vi "ex_BackUpExistFile.vi"(8 "error in":errorcluster, 11 "file path":path) -> (0 "error out":errorcluster, 3 "dup file path":path)   [LabVIEW 2017]
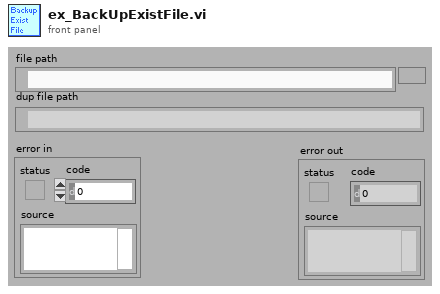
[diagram p1: front panel]
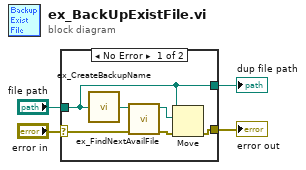
[diagram p0: block diagram]
diagram:
  n1 = case shown="No Error" "error in" {
    selector: "error in" -> [w10 w12]
    tunnel: [w6 w12] -> w3
    tunnel: "file path" -> [w5 w11]
    tunnel: [w5 w11] -> w1
    frame No Error {
      n2 = call <vilib>:"ex_CreateBackupName.vi"("original name"=w5) -> ("backup name"=w9:path)  [unwired: 4 out]
      n3 = call <vilib>:"ex_FindNextAvailFile.vi"("error in"=w10, "desired file path"=w9) -> ("error out"=w8:errorcluster, "next avail file path"=w7:path)  [unwired: 8 out]
      n4 = Move(source path=w5, error in=w8, 10:w7) -> (error out=w6:errorcluster)  [unwired: 4 out]
    }
    frame Error {
    }
  }
  "error out" <- w3
  "dup file path" <- w1
